vi "Sort 2D String Array - StringTransform (Pre Sort).vi"(7 "Input String (\" \")":string) -> (8 "Output String (\" \")":string)   [LabVIEW 2009, in "xijk_select_best_filter.lvlib"]
doc: "Sort 2D String Array - StringTransform (Pre Sort).vi\n\n<B>Description:</B>\n\nThis VI Transforms strings representing numbers or text into strings that will sort properly using the sort 1D array function.\n\nIf the input string represents a number, this VI transforms the string and determines the numeric format string for it. The format string is appended to the input string as a meta tag. \n\nIf the input is a string, this VI determines the lexical class of each character in the string and appends that information to the input string as a meta tag.\n\nAfter sorting, the meta tag is used to transform all of the strings back into their original format.\n\n<B>Usage:</B>\n\nWire all required inputs.\n\n<B>Inputs:</B>\n\nInput String\n- The string to transform.\n\n<B>Outputs:</B>\n\nOutput String\n- This is the output string formatted as a string followed by a meta tag specifying the original format of the input string.\n\n<B>Developed by:</B>\n\nMark Ridgley\nmark.ridgley@logicpd.com"
uses:
  xijk_select_best_filter.lvlib
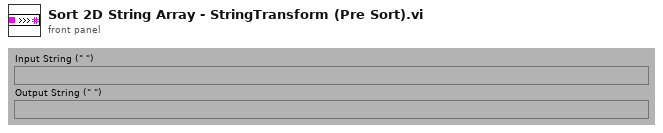
[diagram p1: front panel]
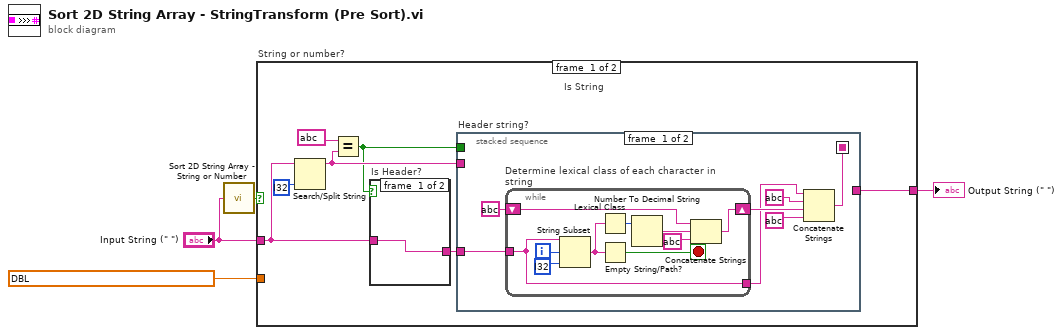
[diagram p0: block diagram]
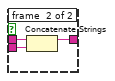
[diagram p3: hidden frame]
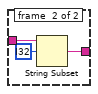
[diagram p4: hidden frame]
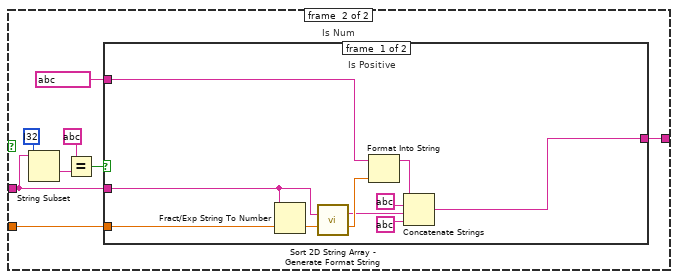
[diagram p5: hidden frame]
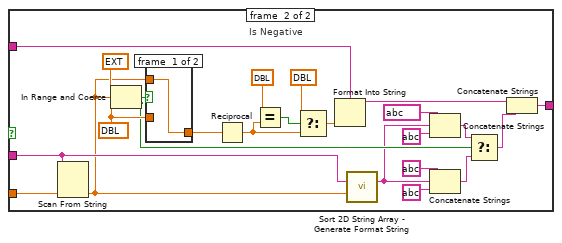
[diagram p6: hidden frame]
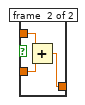
[diagram p7: hidden frame]
diagram:
  n1 = call "Sort 2D String Array - String or Number.vi"("Input String (\" \")"="Input String (\" \")") -> ("Is Num? (F)"=w1:bool)  [unwired: 14 out]
  n2 = case "String or number?" shown="True" w1 {
    tunnel: [w11 w48] -> w4
    tunnel: "Input String (\" \")" -> [w8 w43]
    tunnel: dbl ? ("default (0 dbl)") -> [_ w42]
    frame #0 {
      # "Is String"
      n3 = Search/Split String(string=w8, offset (0)=i32 ?) -> (substring before match=w6:string)  [unwired: 1 in, 2 out]
      n4 = Equal?(x=string ? ("Input String (\" \")"), y=w6) -> (x = y?=w5:bool)
      n5 = case "Is Header?" shown="True" w5 {
        tunnel: w8 -> [w37 w40]
        tunnel: [w37 w38] -> w7
        frame #0 {
        }
        frame #1 {
          n6 = String Subset(string=w40, offset (0)=i32 ?) -> (substring=w38:string)  [unwired: 1 out]
        }
      }
      n7 = stacked-sequence "Header string?" {
        seq-local: [w12 _] -> [_ w31]
        tunnel: w7 -> [w18 _]
        tunnel: [_ w29] -> w11
        tunnel: w6 -> [_ w30]
        tunnel: w5 -> [_ w32]
        frame #0 {
          n8 = while "Determine lexical class of each character in string" {
            tunnel: w18 -> [w25]
            tunnel: [w25] -> w13
            shift-right: [w20] -> w14
            shift-left: string ? -> [w21]
            i -> [w19]
            stop <- w26 stop-if-true
            n9 = String Subset(string=w25, offset (0)=w19, length (rest)=i32 ? ("length (rest)")) -> (substring=w27:string)
            n10 = Lexical Class(1:w27) -> (0:w24:i16)
            n11 = Empty String/Path?(string/path=w27) -> (empty?=w26:bool)
            n12 = Number To Decimal String(number=w24) -> (decimal integer string=w23:string)  [unwired: 1 out]
            n13 = Concatenate Strings(w21, w23, string ? ("string")) -> (w20:string)
          }
          n14 = Concatenate Strings(w13, string ? ("t"), w14, string ? ("Substring")) -> (w12:string)
        }
        frame #1 {
          n15 = case "Is Header?" shown="True" w32 {
            tunnel: w31 -> [w33 w36]
            tunnel: w30 -> [_ w35]
            tunnel: [w33 w34] -> w29
            frame #0 {
            }
            frame #1 {
              n16 = Concatenate Strings(w35, w36) -> (w34:string)
            }
          }
        }
      }
    }
    frame #1 {
      # "Is Num"
      n17 = String Subset(string=w43, length (rest)=i32 ? ("length")) -> (substring=w46:string)  [unwired: 1 out]
      n18 = Equal?(x=string ?, y=w46) -> (x = y?=w44:bool)
      n19 = case shown="True" w44 {
        tunnel: [w55 w73] -> w48
        tunnel: w43 -> [w51 w61]
        tunnel: w42 -> [w54 w63]
        tunnel: string ? ("Format String") -> [w53 w62]
        frame #0 {
          # "Is Positive"
          n20 = Fract/Exp String To Number(string=w51, default (0 dbl)=w54) -> (number=w52:dbl)  [unwired: 3 out]
          n21 = call "Sort 2D String Array - Generate Format String.vi"("Input String (\" \")"=w51, "Number"=w52) -> ("Format String"=w49:string, "Number Out"=w50:dbl)  [unwired: 12 out]
          n22 = Format Into String(format string=w53, w50) -> (resulting string=w56:string)  [unwired: 2 in, 1 out]
          n23 = Concatenate Strings(w56, string ? ("t"), w49, string ? ("Substring")) -> (w55:string)
        }
        frame #1 {
          w71 = dbl ? ("y")
          # "Is Negative"
          n24 = Scan From String(input string=w61, default 1=w63) -> (output 1=w60:dbl)  [unwired: 3 in, 3 out]
          n25 = In Range and Coerce(upper limit=ext ? ("lo"), x=w60, lower limit=w71) -> (In Range?=w64:bool)  [unwired: 1 out]
          n26 = case shown="True" w64 {
            tunnel: w60 -> [w82 w85]
            tunnel: [w82 w84] -> w76
            tunnel: w71 -> [_ w83]
            frame #0 {
            }
            frame #1 {
              n27 = Add(x=w85, y=w83) -> (x+y=w84:dbl)
            }
          }
          n28 = Reciprocal(x=w76) -> (1/x=w77:dbl)
          n29 = Equal?(x=dbl ?, y=w77) -> (x = y?=w80:bool)
          n30 = Select(t=dbl ?, s=w80, f=w77) -> (s? t:f=w79:dbl)
          n31 = Format Into String(format string=w62, w79) -> (resulting string=w72:string)  [unwired: 2 in, 1 out]
          n32 = call "Sort 2D String Array - Generate Format String.vi"("Input String (\" \")"=w61, "Number"=w60) -> ("Format String"=w59:string)  [unwired: 13 out]
          n33 = Concatenate Strings(string ? ("t"), w59, string ? ("Substring")) -> (w69:string)
          n34 = Concatenate Strings(string ? ("t"), w59, string ? ("Substring")) -> (w65:string)
          n35 = Select(t=w69, s=w64, f=w65) -> (s? t:f=w74:string)
          n36 = Concatenate Strings(w72, w74) -> (w73:string)
        }
      }
    }
  }
  "Output String (\" \")" <- w4
